vi "Check Image Analysed.vi"(8 "error in (no error)":errorcluster, 10 "Image Path":path, 11 "DB Path":path) -> (0 "error out":errorcluster, 3 "analysed?":bool)   [LabVIEW 2024]
uses:
  <vilib>/drjdpowell/SQLite Library/SQL Connection/Open (path).vi
  <vilib>/drjdpowell/SQLite Library/SQL Connection/Open (string).vi
  <vilib>/AdvancedString/Path To Command Line String.vi
  <vilib>/drjdpowell/SQLite Library/SQL Connection/Execute SQL (Single Integer).vi
  <vilib>/drjdpowell/SQLite Library/SQL Connection/Connection.lvclass
  <vilib>/drjdpowell/SQLite Library/SQLite.lvlib
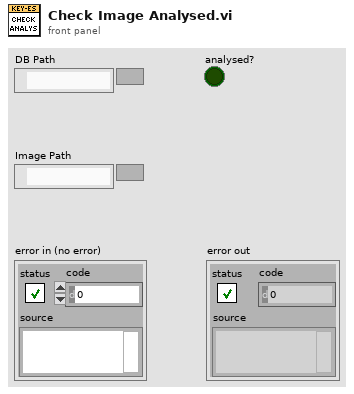
[diagram p1: front panel]
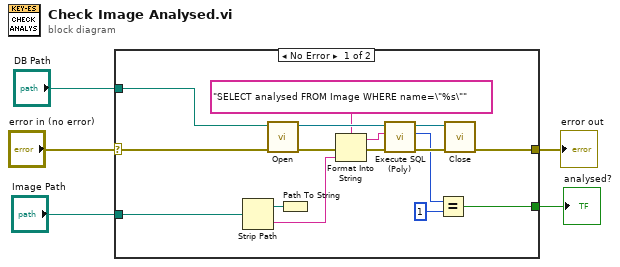
[diagram p0: block diagram]
diagram:
  n1 = case shown="No Error" "error in (no error)" {
    selector: "error in (no error)" -> [w12 w22]
    tunnel: [w14 w22] -> w5
    tunnel: "DB Path" -> [w13 _]
    tunnel: [w7 _] -> w3
    tunnel: "Image Path" -> [w6 _]
    frame No Error {
      n2 = Strip Path(path=w6) -> (stripped path=w11:path, name=w10:string)
      n3 = call-poly <vilib>:"Open.vi"("error in (no error)"=w12, "db file"=w13) -> ("error out"=w21:errorcluster, "SQLite Connection"=w17:refnum<class "Connection.lvclass">)  [unwired: 8 in]
      n4 = Path To String(path=w11) -> ()  [unwired: 1 out]
      n5 = Format Into String(format string="SELECT analysed FROM Image WHERE name=\"%s\"", error in=w21, w10) -> (resulting string=w16:string, error out=w20:errorcluster)  [unwired: 1 in]
      n6 = call-poly <vilib>:"Execute SQL (Poly).vi"("error in (no error)"=w20, "SQL"=w16, "SQLite Connection in"=w17) -> ("error out"=w19:errorcluster, "Result"=w9:i64, "SQLite Connection"=w18:refnum<class "Connection.lvclass">)  [unwired: 6 in]
      n7 = Equal?(x=w9, y=i64 1) -> (x = y?=w7:bool)
      n8 = call-dynamic "Close.vi"("error in (no error)"=w19, "SQLite Connection in"=w18) -> ("error out"=w14:errorcluster)  [unwired: 9 in]
    }
    frame Error {
    }
  }
  "error out" <- w5
  "analysed?" <- w3
